vi "多参标样核查选择对话框.vi"() -> (3 "设置值":T1)   [LabVIEW 2016]
uses:
  <vilib>/Utility/miscctls.llb/LVPointTypeDef.ctl
panel:
  in  "取消按钮":bool
  in  "确定按钮":bool
  in  "叶绿素":bool
  in  "藻密度":bool
  in  "浊度":bool
  in  "电导率":bool
  in  "DO":bool
  in  "pH":bool
  in  "水温":bool
  # "请选择标样核查参数"
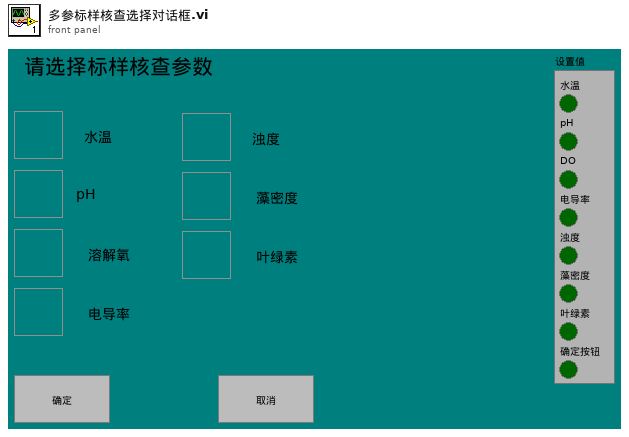
[diagram p1: front panel]
types:
  T1 = cluster{"水温":bool, "pH":bool, "DO":bool, "电导率":bool, "浊度":bool, "藻密度":bool, "叶绿素":bool, "确定按钮":bool}
  T2 = typedef "LVPointTypeDef.ctl" = cluster{"Horizontal":i16, "Vertical":i16}
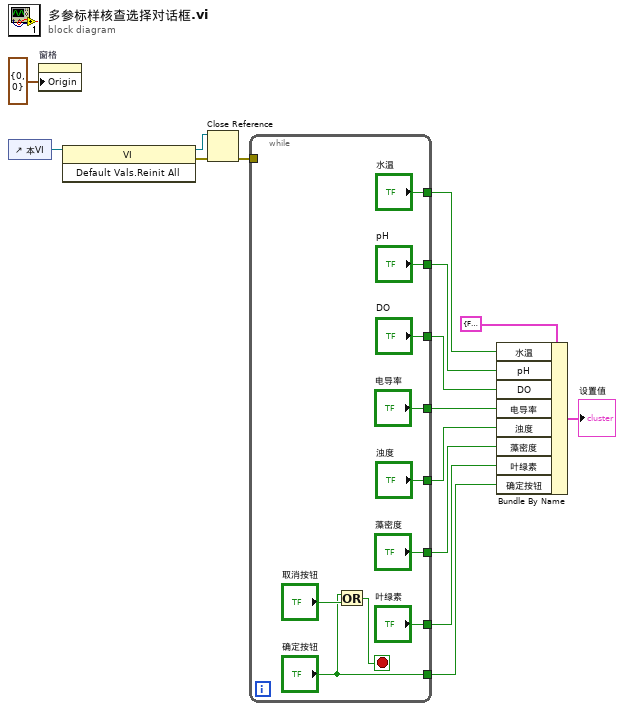
[diagram p0: block diagram]
diagram:
  n1 = control-ref of="本VI"() -> (w4:refnum<vi>)
  n2 = property on="窗格" class="Pane"("Origin"=T2 {"Horizontal"=0, "Vertical"=0} ("原点")) -> ()  [unwired: 2 in, 2 out]
  n3 = invoke class="VI" method="Default Vals.Reinit All"(reference=w4) -> (reference out=w3:refnum<vi>, error out=w2:errorcluster)  [unwired: 2 in, 1 out]
  n4 = Close Reference(reference=w3, error in (no error)=w2) -> (error out=w1:errorcluster)
  n5 = while {
    tunnel: ["水温"] -> w14
    tunnel: ["pH"] -> w13
    tunnel: ["DO"] -> w12
    tunnel: ["电导率"] -> w11
    tunnel: ["浊度"] -> w10
    tunnel: ["藻密度"] -> w9
    tunnel: ["叶绿素"] -> w8
    tunnel: ["确定按钮"] -> w7
    tunnel: w1 -> [_]
    stop <- w24 stop-if-true
    n6 = Or(x="确定按钮", y="取消按钮") -> (x .or. y?=w24:bool)
  }
  n7 = Bundle By Name(cluster=T1 {"水温"=FALSE, "pH"=FALSE, "DO"=FALSE, "电导率"=FALSE, "浊度"=FALSE, "藻密度"=FALSE, "叶绿素"=FALSE, "确定按钮"=FALSE}, "水温"=w14, "pH"=w13, "DO"=w12, "电导率"=w11, "浊度"=w10, "藻密度"=w9, "叶绿素"=w8, "确定按钮"=w7) -> (→"设置值":T1)
